vi "checkNearEnemies.vi"(8 "error in (no error)":errorcluster, 9 "Game":refnum<class "Game.lvclass">, 10 "Robot":refnum<class "Robot.lvclass">, 11 "KickToSkill in":refnum<class "KickToSkill.lvclass">) -> (0 "error out":errorcluster, 2 "canWeakKick":bool, 3 "KickToSkill out":refnum<class "KickToSkill.lvclass">)   [LabVIEW 2020, in "KickToSkill.lvclass"]
uses:
  KickToSkill.lvclass
  Robot_class/Robot.lvclass
  C:/RoboIME/SSL_AI/Object_class/Object.lvclass
  Game_class/Game.lvclass
  Game_class/Game.lvclass/Game.ctl
  Team_class/Team.lvclass/Team.ctl
  Field_class/Field.lvclass/Field.ctl
  Object_class/Object.lvclass/Object.ctl
  Object_class/Read position(x,y).vi
  Game_class/Read FieldRef.vi
  Field_class/Read enemyGoalPosition.vi
  Game_class/Read EnemyRef.vi
  Team_class/Read RobotRef.vi
  Enemy_class/Enemy.lvclass
  C:/RoboIME/SSL_AI/Team_class/Team.lvclass
  Field_class/Field.lvclass
  Utilities_class/Utilities.lvclass
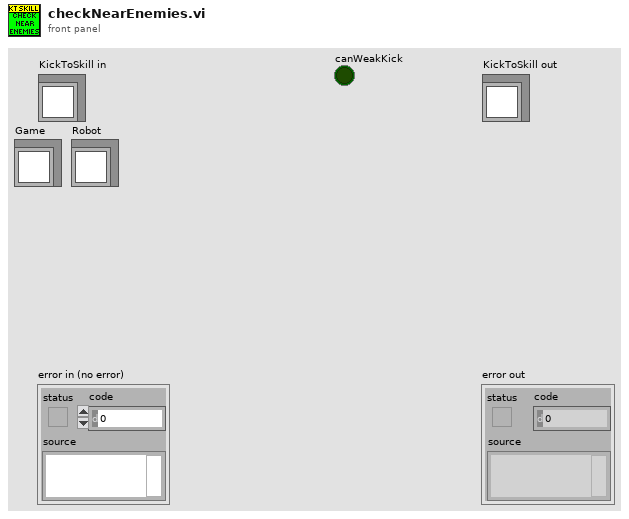
[diagram p1: front panel]
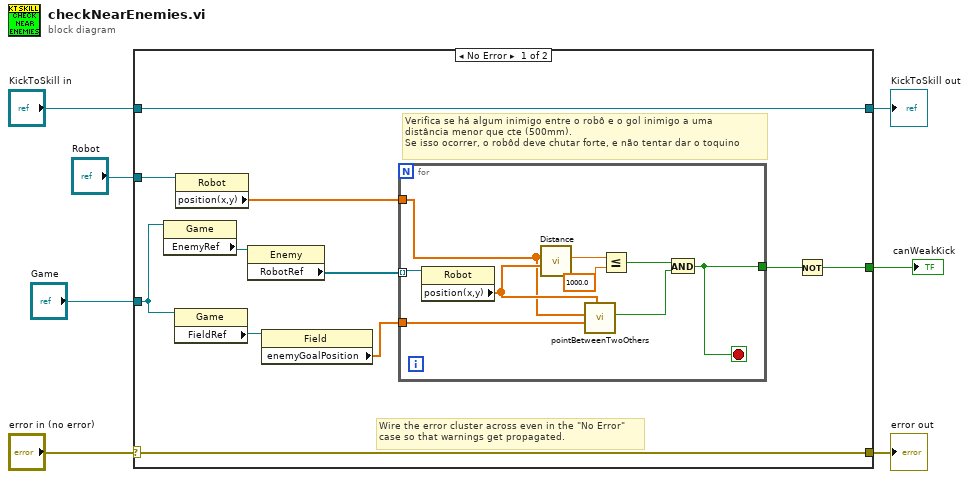
[diagram p0: block diagram]
diagram:
  n1 = case shown="No Error" "error in (no error)" {
    selector: "error in (no error)" -> [w17 w29]
    tunnel: [w17 w29] -> w6
    tunnel: [w18 w28] -> w4
    tunnel: "KickToSkill in" -> [w18 w28]
    tunnel: "Game" -> [w12 _]
    tunnel: "Robot" -> [w14 _]
    tunnel: [w8 _] -> w1
    frame No Error {
      # "Verifica se há algum inimigo entre o robô e o gol inimigo a uma\ndistância menor que cte (500mm).\nSe isso ocorrer, o robôd deve chutar forte, e não tentar dar o toquino"
      # "Wire the error cluster across even in the \"No Error\"\ncase so that warnings get propagated."
      n2 = property class="Game"(reference=w12) -> ("EnemyRef"=w16:refnum<class "Enemy.lvclass">)  [unwired: 1 in, 2 out]
      n3 = property class="Game"(reference=w12) -> ("FieldRef"=w11:refnum<class "Field.lvclass">)  [unwired: 1 in, 2 out]
      n4 = property class="Robot"(reference=w14) -> ("position(x,y)"=w13:dbl[])  [unwired: 1 in, 2 out]
      n5 = property class="Enemy"(reference=w16) -> ("RobotRef"=w15:refnum<class "Robot.lvclass">[])  [unwired: 1 in, 2 out]
      n6 = property class="Field"(reference=w11) -> ("enemyGoalPosition"=w10:dbl[])  [unwired: 1 in, 2 out]
      n7 = for {
        tunnel: w15 -> [w27] mode=indexing
        tunnel: w13 -> [w23]
        tunnel: w10 -> [w22]
        tunnel: [w19] -> w9
        stop <- w19 stop-if-true
        n8 = property class="Robot"(reference=w27) -> ("position(x,y)"=w24:dbl[])  [unwired: 1 in, 2 out]
        n9 = call "Distance.vi"("P1"=w24, "P2"=w23) -> ("Distance"=w26:dbl)  [unwired: 7 in, 2 out]
        n10 = call "pointBetweenTwoOthers.vi"("Q"=w24, "P2"=w22, "P1"=w23) -> ("QBetweenP1P2"=w20:bool)  [unwired: 6 in, 2 out]
        n11 = Less Or Equal?(x=w26, y=1000.0) -> (x <= y?=w21:bool)
        n12 = And(x=w21, y=w20) -> (x .and. y?=w19:bool)
      }
      n13 = Not(x=w9) -> (.not. x?=w8:bool)
    }
    frame Error {
    }
  }
  "error out" <- w6
  "KickToSkill out" <- w4
  "canWeakKick" <- w1
